vi "Write State.vi"(8 "error in (no error)":errorcluster, 10 "State":T1, 11 "Module in":refnum<class "Module.lvclass">) -> (0 "error out":errorcluster, 3 "Module out":refnum<class "Module.lvclass">)   [LabVIEW 2014, in "Module.lvclass"]
uses:
  Module.lvclass
  Module_State.ctl
  Module.lvclass/Module.ctl
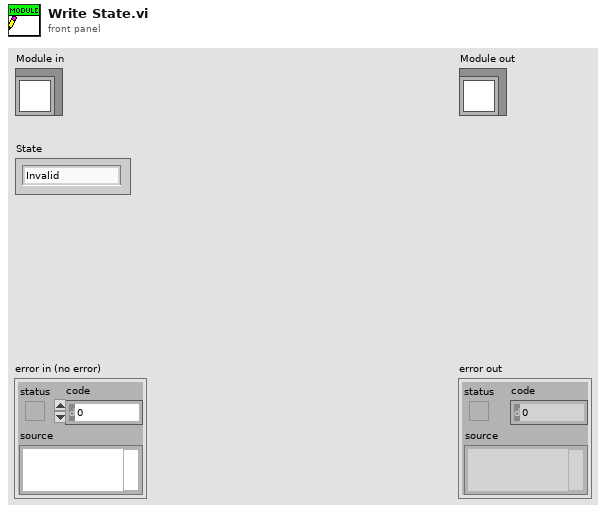
[diagram p1: front panel]
types:
  T1 = typedef "Module.lvclass/Module_State.ctl" = enum16{"Invalid", "Error", "InMemory", "Waiting", "Running"}
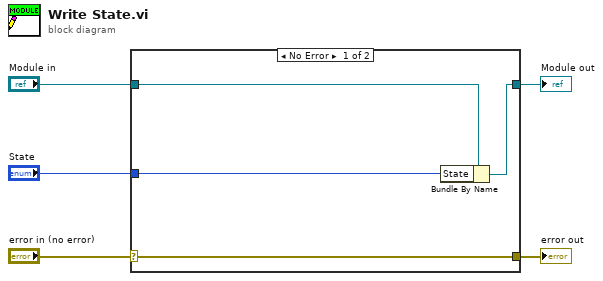
[diagram p0: block diagram]
diagram:
  n1 = case shown="No Error" "error in (no error)" {
    selector: "error in (no error)" -> [w9 w10]
    tunnel: [w9 w10] -> w4
    tunnel: [w7 w11] -> w2
    tunnel: "Module in" -> [w8 w11]
    tunnel: "State" -> [w6 _]
    frame No Error {
      n2 = Bundle By Name(cluster=w8, "State"=w6) -> (w7:refnum<class "Module.lvclass">)
    }
    frame Error {
    }
  }
  "error out" <- w4
  "Module out" <- w2
